vi "Get Status of Ctrl key,Alt key CapsLock key.vi"() -> (0 "capslock":bool, 1 "alt":bool, 2 "ctl":bool, 3 "shift":bool)   [LabVIEW 2012, in "API.lvlib"]
uses:
  API.lvlib
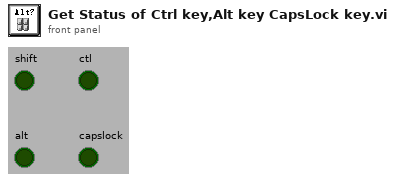
[diagram p1: front panel]
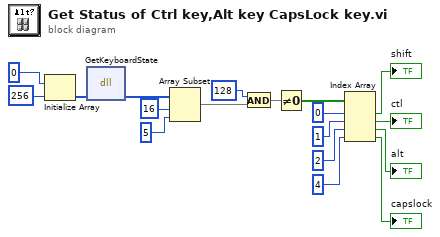
[diagram p0: block diagram]
diagram:
  n1 = Initialize Array(u8 0 ("Element Data"), 256 ("Dimension Size")) -> (w16:u8[])
  n2 = dll-call lib="user32" fn="GetKeyboardState"(w16) -> (w15:u8[])  [unwired: 4 in, 2 out]
  n3 = Array Subset(array=w15, index=16 ("Array Index"), length=5 ("Array Length")) -> (w12:u8[])
  n4 = And(x=u8 128, y=w12) -> (x .and. y?=w10:u8[])
  n5 = Not Equal To 0?(x=w10) -> (x != 0?=w9:bool[])
  n6 = Index Array(array=w9, index #1=0 ("Index"), index #2=1 ("Index"), index #3=2 ("Index"), index #4=4 ("Index")) -> (element #1=→"shift":bool, element #2=→"ctl":bool, element #3=→"alt":bool, element #4=→"capslock":bool)
